vi "Panel.vi"(11 "ColumnPanel in":refnum<class "ColumnPanel.lvclass">) -> ()   [LabVIEW 2020, in "Conditum-Tools.lvlib" / "ColumnPanel.lvclass"]
uses:
  ColumnPanel.lvclass
  C:/Program Files (x86)/National Instruments/LabVIEW 2020/vi.lib/IlluminatedG/IG OOPanel/OOPanel/Panel/Panel.lvclass
  Common Items.ctl
  Accessors.ctl
  Accessor Scope.ctl
  <vilib>/IlluminatedG/IG OOPanel/OOPanel/Panel/Basic UI State.ctl
  ColumnPanel.lvclass/ColumnPanel.ctl
  Conditum-Clone/Columns/Type/Type.lvclass/Type.ctl
  Field Event Data.ctl
  Field Config.ctl
  Conditum-Clone/Columns/Type/Type.lvclass
  <vilib>/Utility/LVClass/Get LV Class Name.vi
  <vilib>/IlluminatedG/IG OOPanel/OOPanel/Panel/Panel.lvclass
  <vilib>/IlluminatedG/IG OOPanel/OOPanel/OOPanel.lvlib
  Conditum-Tools.lvlib
panel:
  out "Type":string
  in  "Common Items":T1
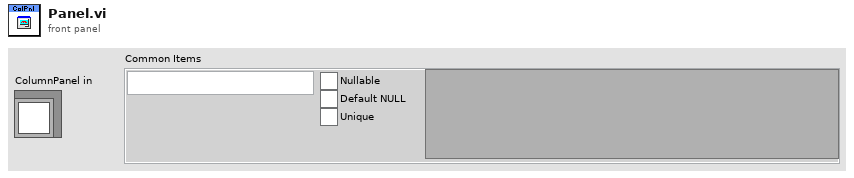
[diagram p1: front panel]
types:
  T1 = typedef "Conditum-Tools.lvlib/ColumnPanel.lvclass/Common Items.ctl" = cluster{"Name":string, "Nullable":bool, "Default NULL":bool, "Unique":bool, "Accessors":T2}
  T2 = typedef "Conditum-Tools.lvlib/Accessors.ctl" = cluster{"Get":T3, "Set":T3}
  T3 = typedef "Conditum-Tools.lvlib/Accessor Scope.ctl" = enum16{"None", "Public", "Protected", "Private"}
  T4 = typedef "OOPanel.lvlib/Panel.lvclass/Basic UI State.ctl" = enum16{"Init", "Run", "Close"}
  T5 = typedef "Conditum-Tools.lvlib/ColumnPanel.lvclass/Field Event Data.ctl" = cluster{"Field Config":T6}
  T6 = typedef "Conditum-Tools.lvlib/Field Config.ctl" = cluster{"Type":refnum<class "Type.lvclass">, "Accessors":T2}
  T7 = typedef "Conditu2.lvlib/Field Type.ctl" = enum16{"None", "ID", "Boolean", "Integer", "Double", "Timestamp", "String", "Text", "Entity"}
  T8 = typedef "Conditum-Tools.lvlib/ColumnPanel.lvclass/Events.ctl" = cluster{"Update":refnum<user-event>, "Value":refnum<user-event>, "Valid":refnum<user-event>, "Highlight":refnum<user-event>, "Property Update":refnum<user-event>}
  T9 = typedef "OOPanel.lvlib/Panel.lvclass/Panel Events.ctl" = cluster{"Visbility":refnum<user-event>, "Close":refnum<user-event>}
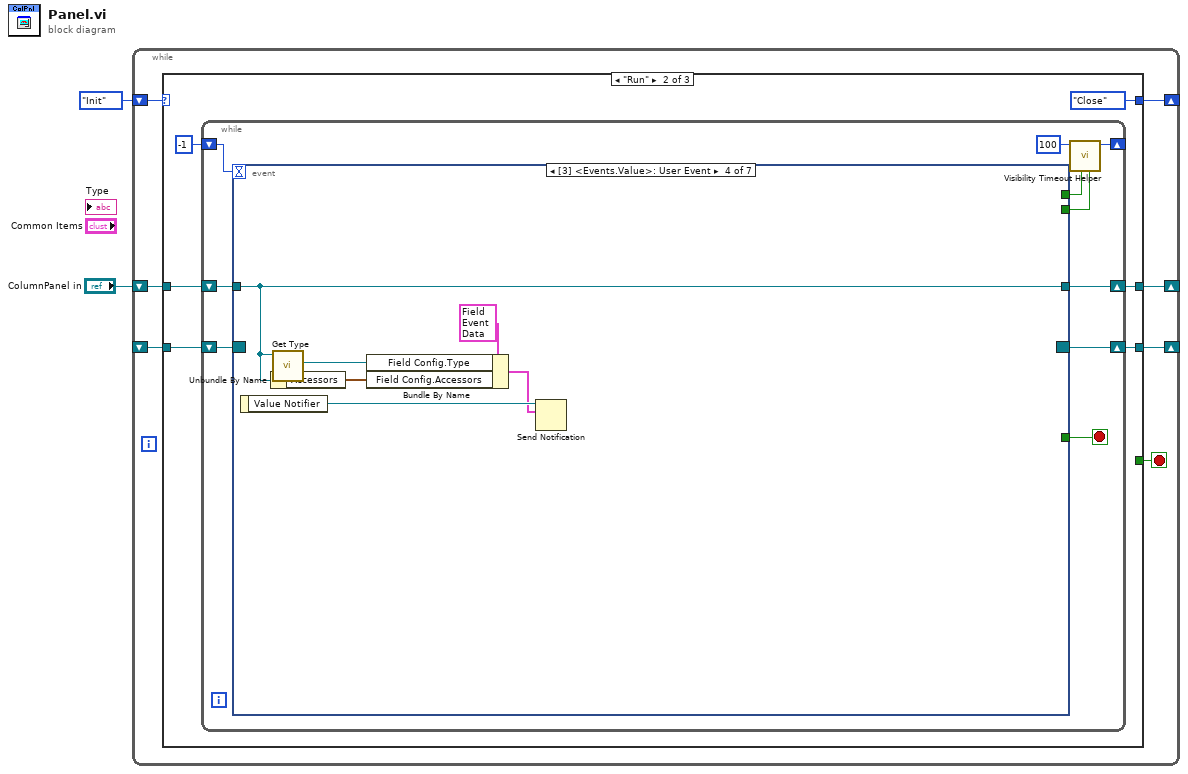
[diagram p0: block diagram]
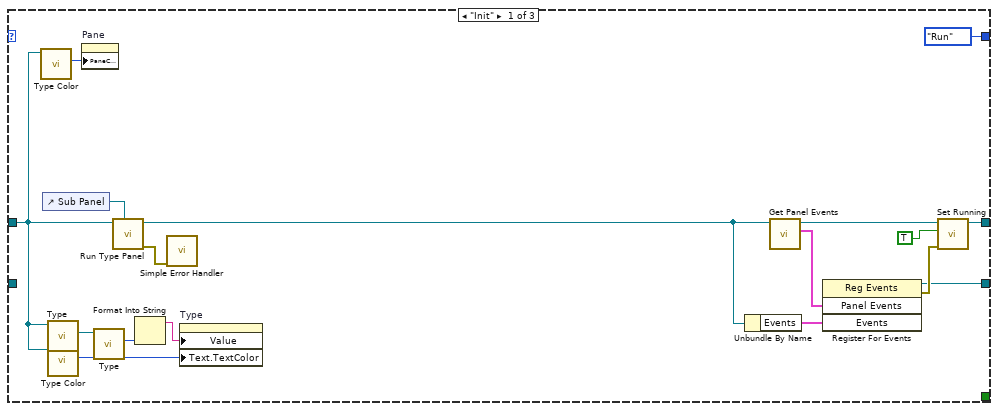
[diagram p2: hidden frame]
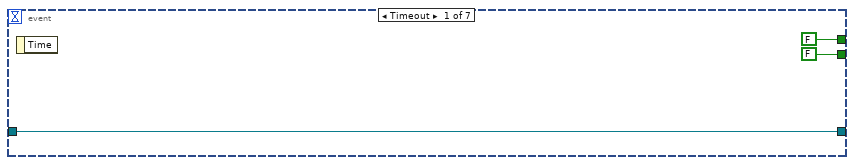
[diagram p3: hidden frame]
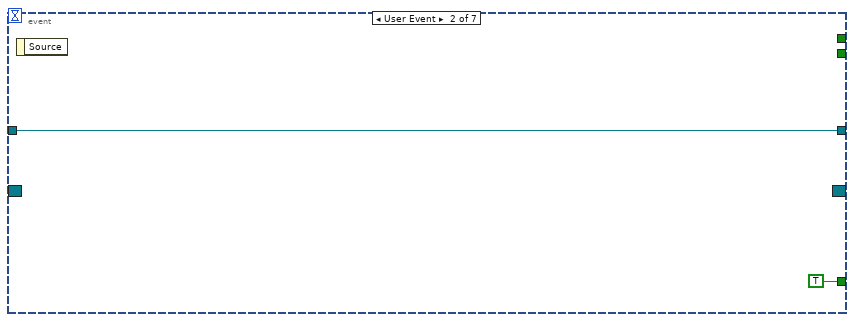
[diagram p4: hidden frame]
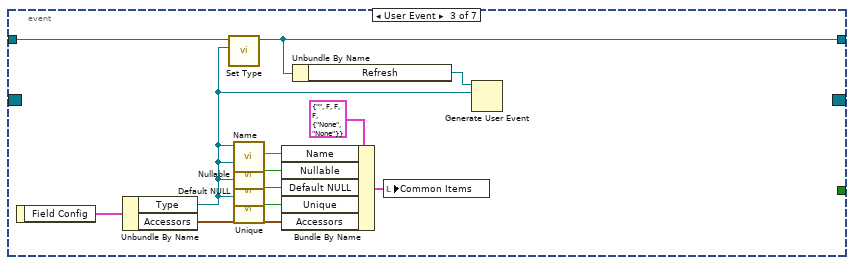
[diagram p5: hidden frame]
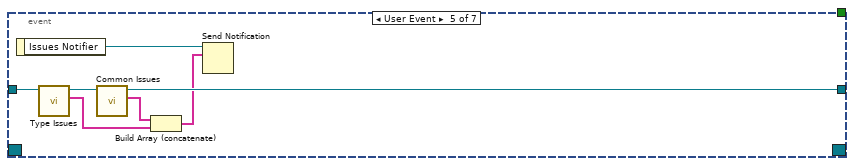
[diagram p6: hidden frame]
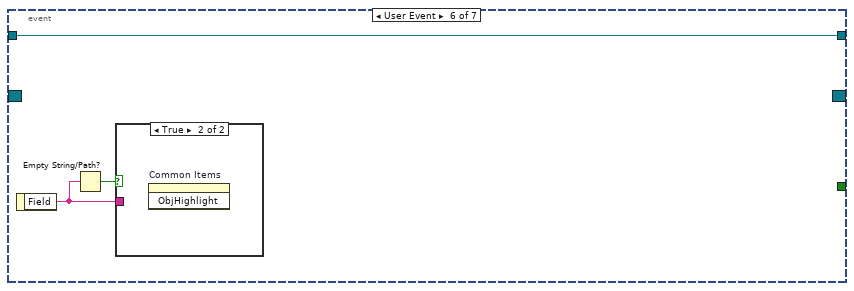
[diagram p7: hidden frame]
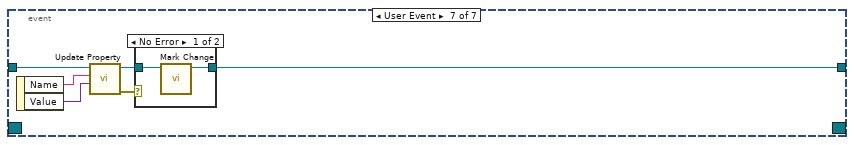
[diagram p9: hidden frame]
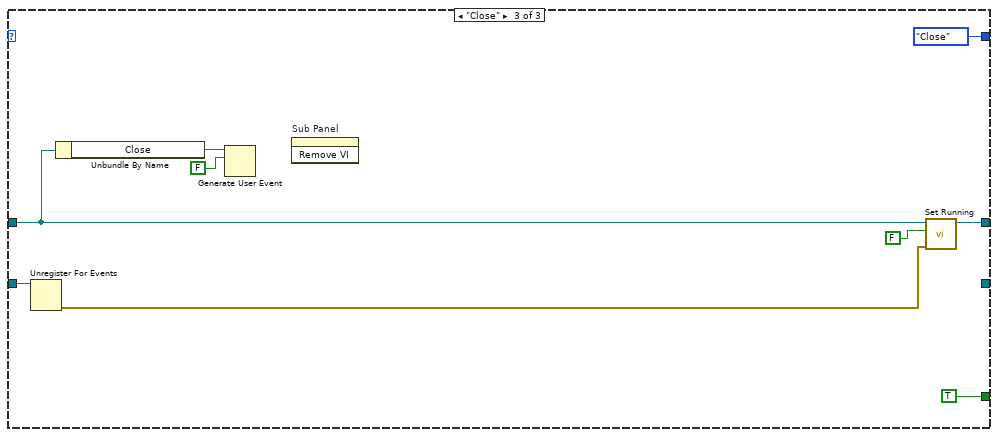
[diagram p11: hidden frame]
diagram:
  n1 = while {
    shift-right: [w8] -> _
    shift-left: _ -> [w9]
    shift-right: [w6] -> _
    shift-left: Basic_UI_State."Init" ("Basic UI State") -> [w7]
    shift-right: [w4] -> _
    shift-left: "ColumnPanel in" -> [w3]
    stop <- w5 stop-if-true
    n2 = case shown="\"Run\"" w7 {
      tunnel: w9 -> [_ w32 w89]
      tunnel: [w23 w30 _] -> w8
      tunnel: [Basic_UI_State."Run" ("Basic UI State") Basic_UI_State."Close" ("Basic UI State") Basic_UI_State."Close" ("Basic UI State")] -> w6
      tunnel: [_ _ TRUE] -> w5
      tunnel: [w22 w27 w88] -> w4
      tunnel: w3 -> [w14 w28 w87]
      frame "Init" {
        n3 = call-dynamic "Type Color.vi"("ColumnPanel in"=w14) -> ("Type Color"=w18:u32)  [unwired: 10 in]
        n4 = control-ref of="Sub Panel"() -> (w17:refnum<vi>)
        n5 = call-dynamic "Type.vi"("ColumnPanel in"=w14) -> ("Type"=w13:refnum<class "Type.lvclass">)  [unwired: 10 in]
        n6 = call-dynamic "Type Color.vi"("ColumnPanel in"=w14) -> ("Type Color"=w11:u32)  [unwired: 10 in]
        n7 = property on="Pane" class="Pane"("PaneColor"=w18) -> ()  [unwired: 2 in, 2 out]
        n8 = call "Type.vi"("Type in"=w13) -> ("Type"=w12:T7)  [unwired: 10 in]
        n9 = call "Run Type Panel.vi"("Sub Panel"=w17, "ColumnPanel in"=w14) -> ("error out"=w16:errorcluster, "ColumnPanel out"=w15:refnum<class "ColumnPanel.lvclass">)  [unwired: 8 in]
        n10 = Format Into String(w12) -> (resulting string=w10:string)  [unwired: 3 in, 1 out]
        n11 = call <vilib>:"Simple Error Handler.vi"("error in (no error)"=w16) -> ()  [unwired: 4 in, 5 out]
        n12 = property on="Type" class="Str"("Value"=w10, "Text.TextColor"=w11) -> ()  [unwired: 2 in, 2 out]
        n13 = Unbundle By Name(w15) -> ("Events"=w19:T8)
        n14 = call <vilib>:"Get Panel Events.vi"("Panel in"=w15) -> ("Panel Events"=w20:T9, "Panel out"=w21:refnum<class "ColumnPanel.lvclass">)  [unwired: 8 in, 1 out]
        n15 = register-events(w20, w19) -> (reference out=w23:refnum<event-registration>, error out=w25:errorcluster)  [unwired: 2 in]
        n16 = call <vilib>:"Set Running.vi"("error in (no error)"=w25, "Running"=TRUE, "Panel in"=w21) -> ("Panel out"=w22:refnum<class "ColumnPanel.lvclass">)  [unwired: 7 in, 1 out]
      }
      frame "Run" {
        n17 = while {
          shift-right: [w38] -> w30
          shift-left: w32 -> [w39]
          shift-right: [w41] -> _
          shift-left: -1 ("Timeout") -> [w40]
          shift-right: [w33] -> w27
          shift-left: w28 -> [w34]
          stop <- w35 stop-if-true
          n18 = event shown="[3] <Events.Value>: User Event" {
            selector: w39 -> [_ _ _ _ _ _ _]
            dyn-events: [_ _ _ _ _ _ _] -> w38
            timeout: w40 -> [_ _ _ _ _ _ _]
            tunnel: [FALSE _ _ _ _ _ _] -> w37
            tunnel: [FALSE _ _ _ _ _ _] -> w36
            tunnel: [_ TRUE _ _ _ _ _] -> w35
            tunnel: w34 -> [w43 w46 w58 w62 w71 w75 w81]
            tunnel: [w43 w46 w48 w62 w67 w75 w76] -> w33
            event Timeout {
              n19 = event-data() -> ()  [unwired: 1 in, 1 out]
            }
            event User Event {
              n20 = event-data() -> ()  [unwired: 1 in, 1 out]
            }
            event User Event {
              n21 = event-data() -> ("Field Config"=w59:T6)  [unwired: 1 in]
              n22 = Unbundle By Name(w59) -> ("Type"=w49:refnum<class "Type.lvclass">, "Accessors"=w55:T2)
              n23 = call-dynamic "Set Type.vi"("Type"=w49, "ColumnPanel in"=w58) -> ("ColumnPanel out"=w48:refnum<class "ColumnPanel.lvclass">)  [unwired: 9 in]
              n24 = call "Name.vi"("Type in"=w49) -> ("Table Name"=w54:string)  [unwired: 10 in]
              n25 = call "Nullable.vi"("Type in"=w49) -> ("Nullable"=w52:bool)  [unwired: 10 in]
              n26 = call "Default NULL.vi"("Type in"=w49) -> ("Default NULL"=w51:bool)  [unwired: 10 in]
              n27 = call "Unique.vi"("Type in"=w49) -> ("Unique"=w50:bool)  [unwired: 10 in]
              n28 = Bundle By Name(cluster=T1 {"Name"="", "Nullable"=FALSE, "Default NULL"=FALSE, "Unique"=FALSE, "Accessors"={"Get"=enum."None", "Set"=enum."None"}} ("Common Items"), "Name"=w54, "Nullable"=w52, "Default NULL"=w51, "Unique"=w50, "Accessors"=w55) -> (w53:T1)
              n29 = Unbundle By Name(w48) -> ("Refresh"=w57:refnum<user-event>)
              n30 = local write "Common Items"(w53) -> ()
              n31 = Generate User Event(user event=w57, event data cluster=w49) -> ()  [unwired: 2 in, 2 out]
            }
            event User Event {
              n32 = event-data() -> ("Value Notifier"=w65:refnum<notifier>)  [unwired: 1 in]
              n33 = Unbundle By Name(w62) -> ("Accessors"=w61:T2)
              n34 = call-dynamic "Get Type.vi"("ColumnPanel in"=w62) -> ("Type"=w60:refnum<class "Type.lvclass">)  [unwired: 10 in]
              n35 = Bundle By Name(cluster=T5 {"Field Config"={"Type"=refnum, "Accessors"={"Get"=enum."None", "Set"=enum."None"}}} ("notification"), "Field Config.Type"=w60, "Field Config.Accessors"=w61) -> (w63:T5)
              n36 = Send Notification(notification=w63, notifier=w65) -> ()  [unwired: 1 in, 2 out]
            }
            event User Event {
              n37 = event-data() -> ("Issues Notifier"=w72:refnum<notifier>)  [unwired: 1 in]
              n38 = call-dynamic "Type Issues.vi"("ColumnPanel in"=w71) -> ("Issues"=w69:string[], "ColumnPanel out"=w70:refnum<class "ColumnPanel.lvclass">)  [unwired: 8 in, 1 out]
              n39 = call "Common Issues.vi"("ColumnPanel in"=w70) -> ("Issues"=w68:string[], "ColumnPanel out"=w67:refnum<class "ColumnPanel.lvclass">)  [unwired: 8 in, 1 out]
              n40 = Build Array (concatenate)(w68, w69) -> (w66:string[])
              n41 = Send Notification(notification=w66, notifier=w72) -> ()  [unwired: 1 in, 2 out]
            }
            event User Event {
              n42 = event-data() -> ("Field"=w73:string)  [unwired: 1 in]
              n43 = Empty String/Path?(string/path=w73) -> (empty?=w74:bool)
              n44 = case shown="True" w74 {
                tunnel: w73 -> [_ _]
                frame False {
                }
                frame True {
                  n45 = invoke on="Common Items" class="Clust (strict)" method="ObjHighlight"() -> ()  [unwired: 3 in, 3 out]
                }
              }
            }
            event User Event {
              n46 = event-data() -> ("Name"=w80:string, "Value"=w79:variant)  [unwired: 1 in]
              n47 = call-dynamic "Update Property.vi"("Value"=w79, "Name"=w80, "ColumnPanel in"=w81) -> ("error out"=w77:errorcluster, "ColumnPanel out"=w78:refnum<class "ColumnPanel.lvclass">)  [unwired: 7 in]
              n48 = case shown="No Error" w77 {
                tunnel: w78 -> [w83 w84]
                tunnel: [w82 w84] -> w76
                frame No Error {
                  n49 = call "Mark Change.vi"("ColumnPanel in"=w83) -> ("ColumnPanel out"=w82:refnum<class "ColumnPanel.lvclass">)  [unwired: 10 in]
                }
                frame Error {
                }
              }
            }
          }
          n50 = call <vilib>:"Visibility Timeout Helper.vi"("Update?"=w36, "Use Timeout?"=w37, "Visible Timeout mS"=100) -> ("Timeout"=w41:i32)  [unwired: 8 in]
        }
      }
      frame "Close" {
        n51 = Unregister For Events(event registration refnum=w89) -> (error out=w91:errorcluster)  [unwired: 1 in]
        n52 = Unbundle By Name(w87) -> ("Close"=w86:refnum<user-event>)
        n53 = Generate User Event(user event=w86, event data cluster=FALSE ("event data")) -> ()  [unwired: 2 in, 2 out]
        n54 = invoke on="Sub Panel" class="SubPnl" method="Remove VI"() -> ()  [unwired: 3 in, 3 out]
        n55 = call <vilib>:"Set Running.vi"("error in (no error)"=w91, "Running"=FALSE, "Panel in"=w87) -> ("Panel out"=w88:refnum<class "ColumnPanel.lvclass">)  [unwired: 7 in, 1 out]
      }
    }
  }
